vi "Json_Data_Path_Python.vi"(0 "Json File Path":path, 7 "Multiple Read":T2 {"ERD Number" format="%x"}, 11 "error in":errorcluster) -> (8 "Multiple Read 2":T1[](array[typedef]) {"ERD Number" format="%x"}, 15 "error out":errorcluster)   [LabVIEW 2021]
uses:
  Controles/Multiple_Read_ERD.ctl
  Controles/Read_ERD.ctl
  <vilib>/JDP Science/JSONtext/String Subset.vi
  <vilib>/JDP Science/JSONtext/support/Strip Quotes and Unescape.vi
  <vilib>/JDP Science/JSONtext/support/Unescape JSON string.vi
  <vilib>/JDP Science/JSONtext/Parsing/Parse Full Path or Item Name.vi
  <vilib>/JDP Science/JSONtext/Offset/Find Item Locations by Path.vi
  <vilib>/JDP Science/JSONtext/JSONtext.lvlib
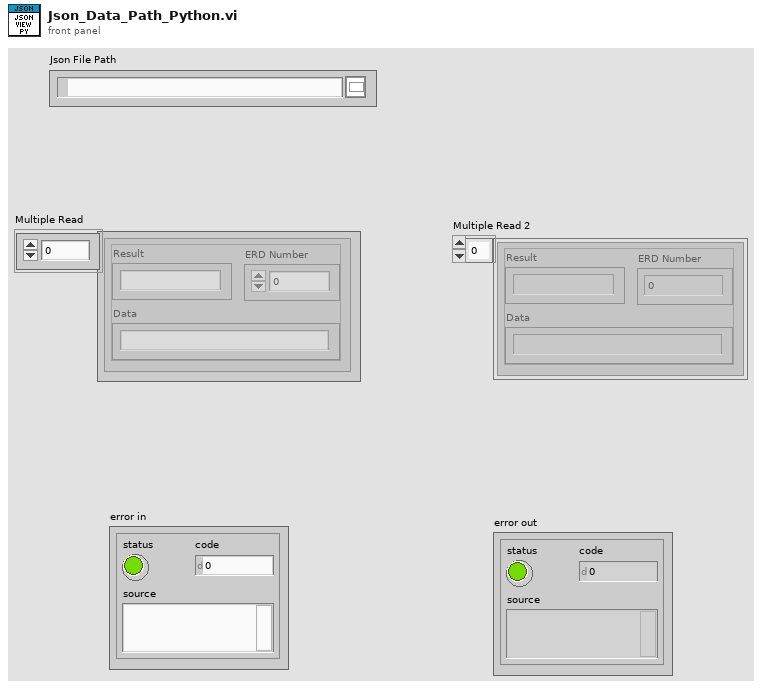
[diagram p1: front panel]
types:
  T1 = typedef "Read_ERD.ctl" = cluster{"Result":string, "ERD Number":i64, "Data":string}
  T2 = typedef "Multiple_Read_ERD.ctl" = T1[]
  T3 = enum16{"open", "replace", "create", "open or create", "replace or create", "replace or create with confirmation"}
  T4 = cluster{"Multiple Read[0]":T1, "Multiple Read[1]":T1, "Multiple Read[2]":T1, "Multiple Read[3]":T1, "Multiple Read[4]":T1, "Multiple Read[5]":T1, "Multiple Read[6]":T1, "Multiple Read[7]":T1, "Multiple Read[8]":T1}
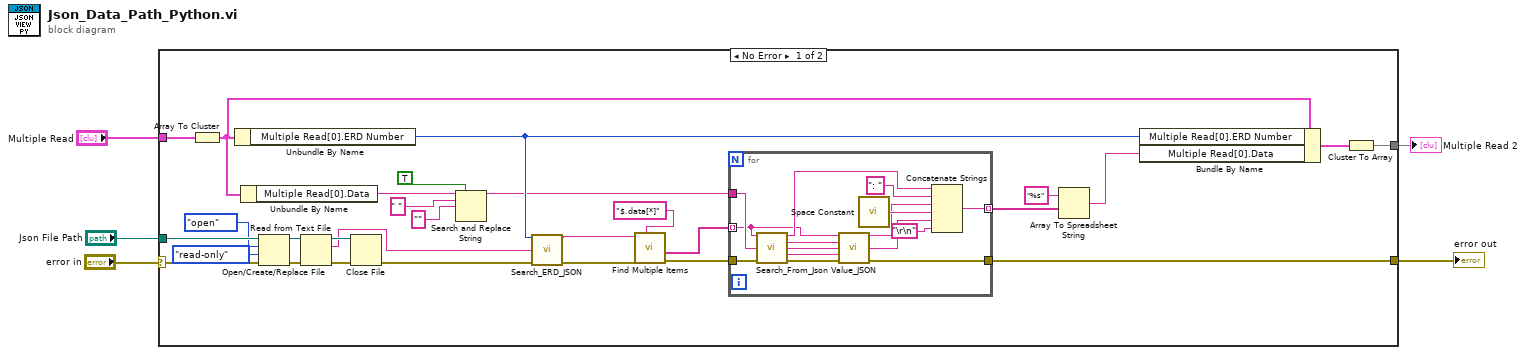
[diagram p0: block diagram]
diagram:
  n1 = case shown="No Error" "error in" {
    selector: "error in" -> [w18 w50]
    tunnel: [w9 w50] -> w4
    tunnel: "Json File Path" -> [w30 _]
    tunnel: "Multiple Read" -> [w29 _]
    tunnel: [w28 _] -> w1
    frame No Error {
      n2 = Array To Cluster(array=w29) -> (cluster=w8:T4)
      n3 = Unbundle By Name(w8) -> ("Multiple Read[0].ERD Number"=w14:i64)
      n4 = Unbundle By Name(w8) -> ("Multiple Read[0].Data"=w22:string)
      n5 = Open/Create/Replace File(file path (use dialog)=w30, error in=w18, operation (0:open)=T3."open", access (0:read/write)=enum16{"read/write", "read-only", "write-only"}."read-only") -> (refnum out=w32:refnum<file>, error out=w34:errorcluster)  [unwired: 2 in, 1 out]
      n6 = Read from Text File(file (use dialog)=w32, error in=w34) -> (refnum out=w31:refnum<file>, text=w11:string, error out=w33:errorcluster)  [unwired: 2 in, 1 out]
      n7 = Close File(refnum=w31, error in=w33) -> (error out=w12:errorcluster)  [unwired: 1 out]
      n8 = Search and Replace String(replace all?=TRUE ("replace all? (F)"), input string=w22, search string=" ", replace string="" ("replace string (\"\")")) -> (result string=w10:string)  [unwired: 4 in, 3 out]
      n9 = call "Search_ERD_JSON.vi"("ERD Number"=w14, "JSON Text"=w11, "error in"=w12) -> ("ERD"=w15:string, "error out"=w16:errorcluster)  [unwired: 11 in]
      n10 = call <vilib>:"Find Multiple Items.vi"("$Path or Item Name"="$.data[*]", "error in (no error)"=w16, "JSON"=w15) -> ("error out"=w13:errorcluster, "<JSON>"=w26:string[])  [unwired: 5 in, 2 out]
      n11 = for {
        tunnel: w26 -> [w43] mode=indexing
        tunnel: w10 -> [w45]
        tunnel: [w47] -> w20 mode=indexing
        tunnel: [w36] -> w9
        tunnel: w13 -> [w35]
        n12 = call "Search_From_Json.vi"("Data JSON"=w43, "ERD"=w45, "error in"=w35) -> ("Name"=w44:string, "Type"=w42:string, "Size data"=w41:string, "Hexa"=w40:string, "error IO"=w39:errorcluster)  [unwired: 8 in]
        n13 = call "Value_JSON.vi"("Data JSON"=w43, "Type"=w42, "Size data"=w41, "Hexa"=w40, "error in"=w39) -> ("Value_string"=w38:string, "Hexa value"=w37:string, "error IO"=w36:errorcluster)  [unwired: 8 in]
        n14 = call <vilib>:"Space Constant.vi"() -> ("String"=w48:string)
        n15 = Concatenate Strings(w44, ": " ("string"), w38, w48, w37, "\r\n") -> (w47:string)
      }
      n16 = Array To Spreadsheet String(array=w20, 3:"%s" ("format string")) -> (spreadsheet string=w19:string)  [unwired: 1 in]
      n17 = Bundle By Name(cluster=w8, "Multiple Read[0].ERD Number"=w14, "Multiple Read[0].Data"=w19) -> (w17:T4)
      n18 = Cluster To Array(cluster=w17) -> (array=w28:T1[])
    }
    frame Error {
    }
  }
  "error out" <- w4
  "Multiple Read 2" <- w1
